vi "2D experiment mouse.vi"() -> ()   [LabVIEW 2011]
uses:
  <vilib>/Platform/TimedLoop/XDataNode/timing_clust.ctl
  <vilib>/Platform/TimedLoop/XDataNode/nitl_modes.ctl
  <vilib>/Platform/TimedLoop/XDataNode/wakeup.ctl
  <vilib>/Utility/cursorutil.llb/Set Cursor (Cursor ID).vi
  <vilib>/Utility/inputDevices.llb/closeMouse.vi
  <vilib>/Utility/inputDevices.llb/mouseAcquire.vi
  <vilib>/Utility/file.llb/Write To Spreadsheet File (DBL).vi
  <vilib>/Utility/file.llb/Write To Spreadsheet File (I64).vi
  <vilib>/Platform/TimedLoop/XDataNode/XDataNode.xnode
  User32.dll
  <vilib>/Platform/TimedLoop/XDataNode/XDNodeRunTimeDep.lvlib
panel:
  out "initial time":u32
  out "XY Graph":cluster{"Y":dbl[], "Y":dbl[]}[](graph)
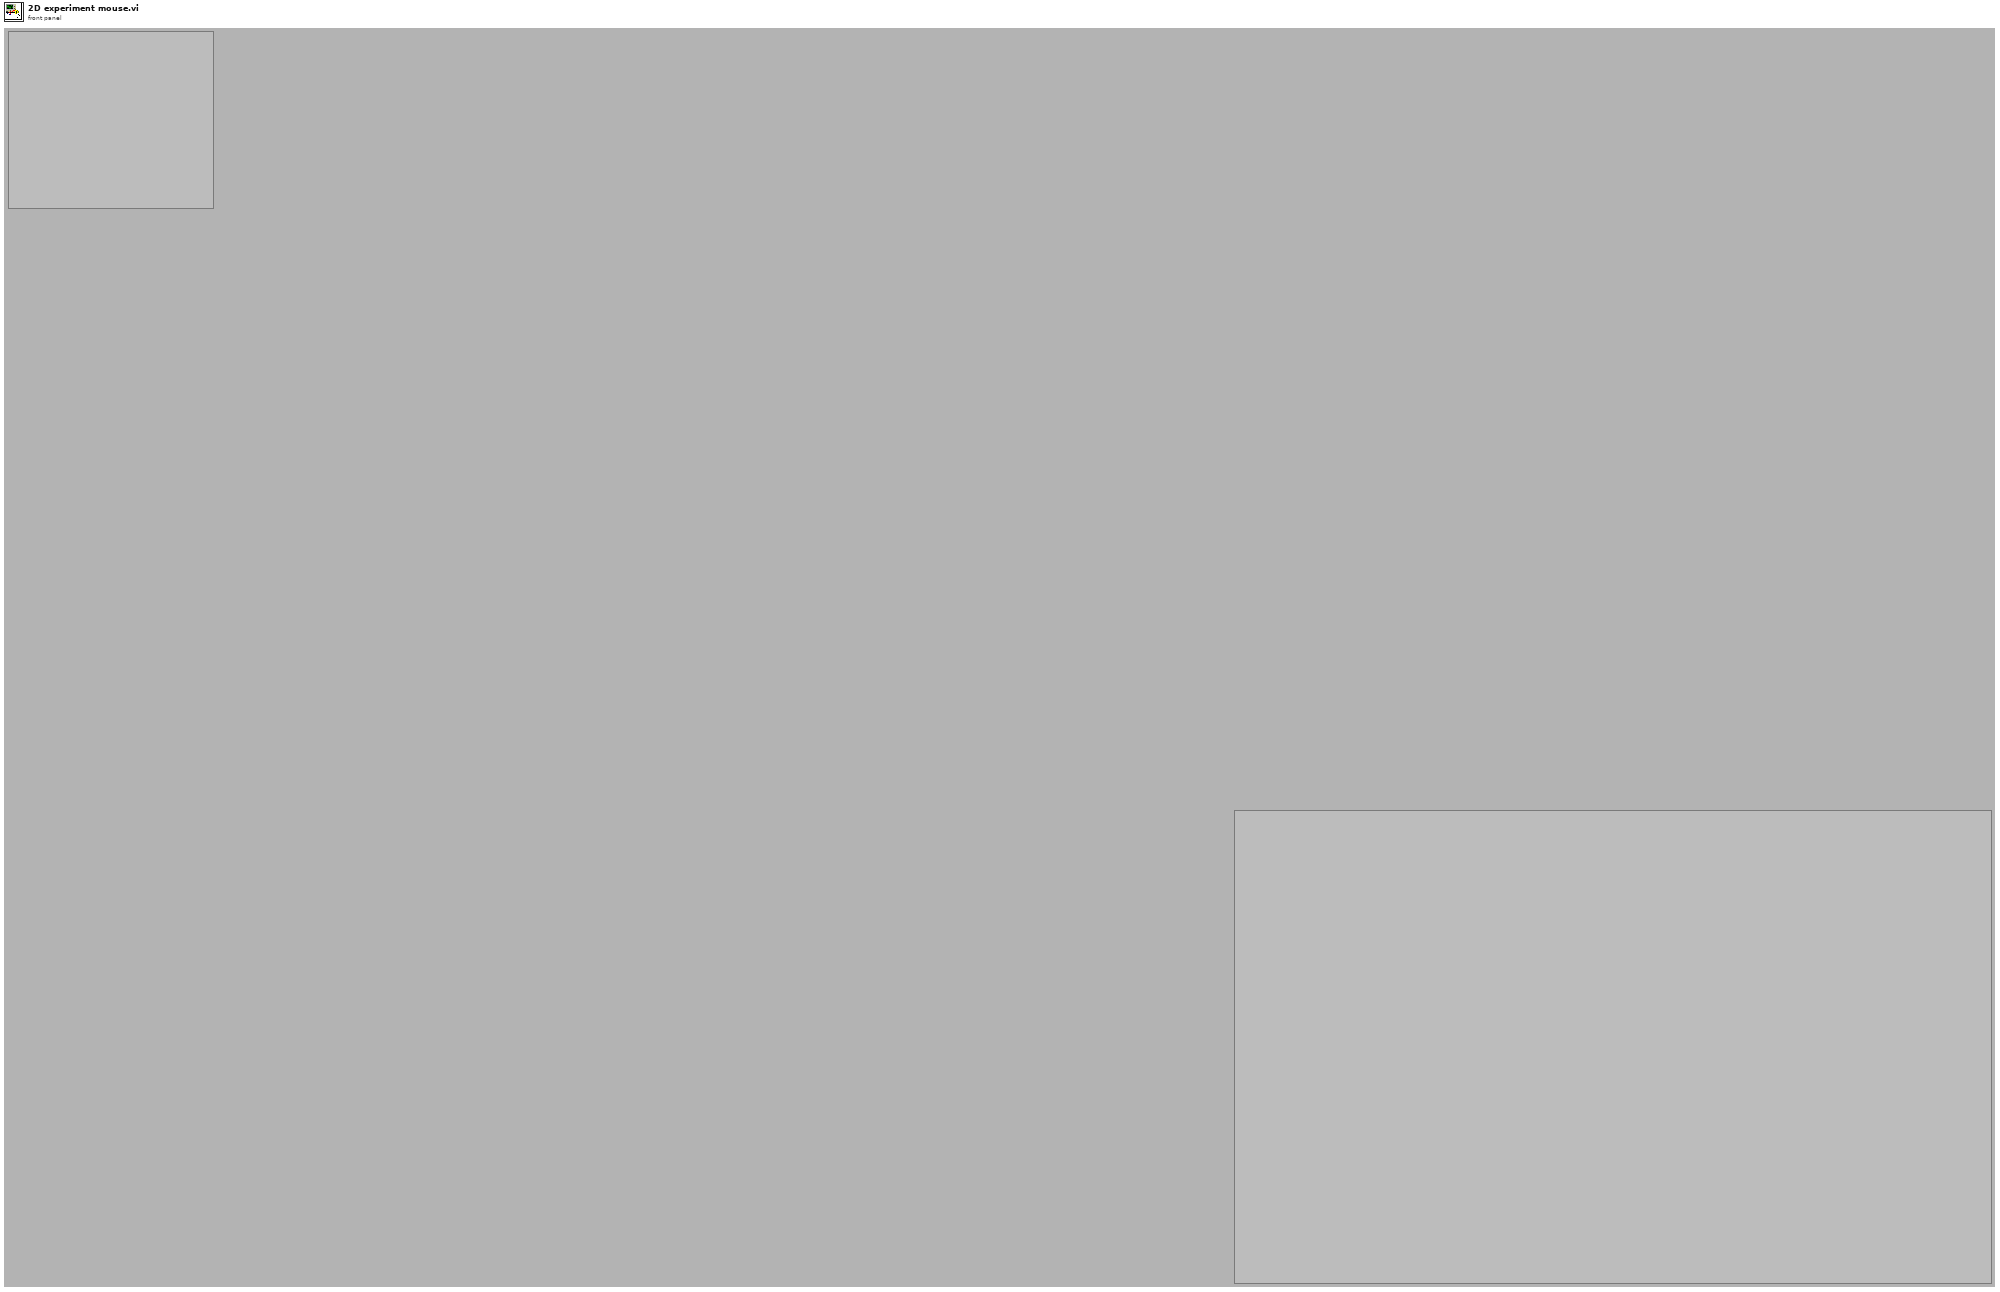
[diagram p1: front panel]
types:
  T1 = enum16{"open", "replace", "create", "open or create", "replace or create", "replace or create with confirmation"}
  T2 = typedef "XDNodeRunTimeDep.lvlib/timing_clust.ctl" = cluster{"Expected End [f-1]":u64, "Actual End [f-1]":u64, "Finished Late? [f-1]":bool, "Expected End [i-1]":u64, "Actual End [i-1]":u64, "Finished Late? [i-1]":bool, "Expected Start [i]":u64, "Actual Start [i]":u64, "Expected Start [f]":u64, "Actual Start [f]":u64, "Source Name":string, "Structure Name":string, "Period":i64, "Deadline":i64, "Offset":i64, "Start":i64, "Priority":i32, "Timeout":i32, "Mode":T3, "Wakeup Reason":T4, "Error":errorcluster, "Source Type":string, "Secondary Source Type":string, "Global End Time":u64, "Global Start Time":u64, "Frame Duration":u64, "Iteration Duration":u64, "Assigned CPU":i32, "I/O Scan Engine Mode":u32}
  T3 = typedef "XDNodeRunTimeDep.lvlib/nitl_modes.ctl" = enum32{"No Change", "Process missed periods, maintain original phase", "Discard missed periods, maintain original phase", "Process missed periods, ignore original phase", "Discard missed periods, ignore original phase"}
  T4 = typedef "XDNodeRunTimeDep.lvlib/wakeup.ctl" = enum32{"Normal", "Aborted", "Asynchronous wakeup", "Timing source error", "Timed loop error", "Timeout"}
  T5 = typedef "LVAllMonitorsDisplayTypeDef.ctl" = cluster{"Bounds":cluster{"Left":i16, "Top":i16, "Right":i16, "Bottom":i16}, "Depth":i16}[]
  T6 = cluster{"Bounds":cluster{"Left":i16, "Top":i16, "Right":i16, "Bottom":i16}, "Depth":i16}
  T7 = cluster{"Left":i16, "Top":i16, "Right":i16, "Bottom":i16}
  T8 = cluster{"Horizontal":i32, "Vertical":i32, "Scrolling":i32}
  T9 = cluster{"button 1":bool, "button 2":bool, "button 3":bool, "button 4":bool}
  T10 = cluster{"Radius":dbl, "x0":dbl, "y0":dbl, "D":dbl, bool}
  T11 = typedef "LVPoint32TypeDef.ctl" = cluster{"Horizontal":i32, "Vertical":i32}
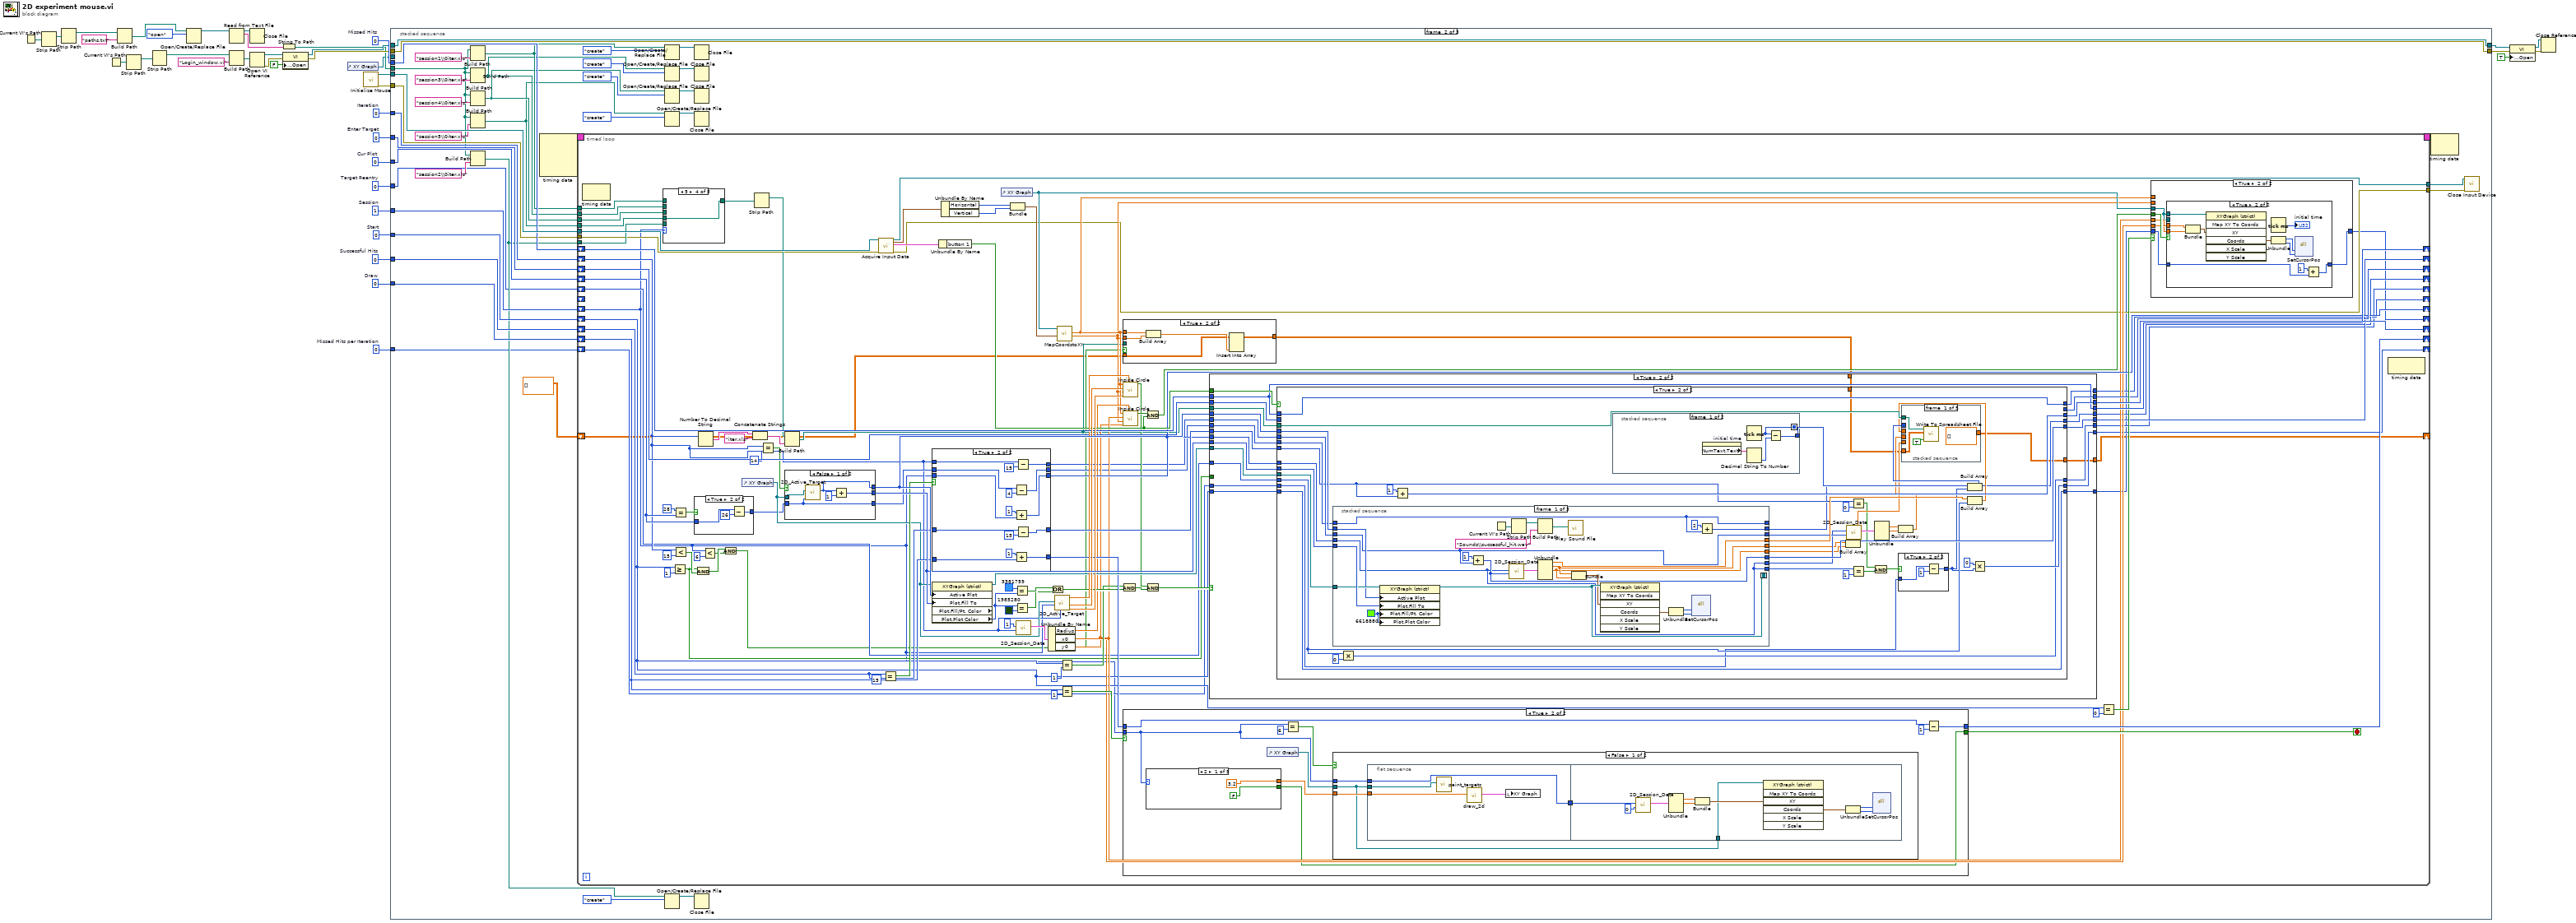
[diagram p0: block diagram]
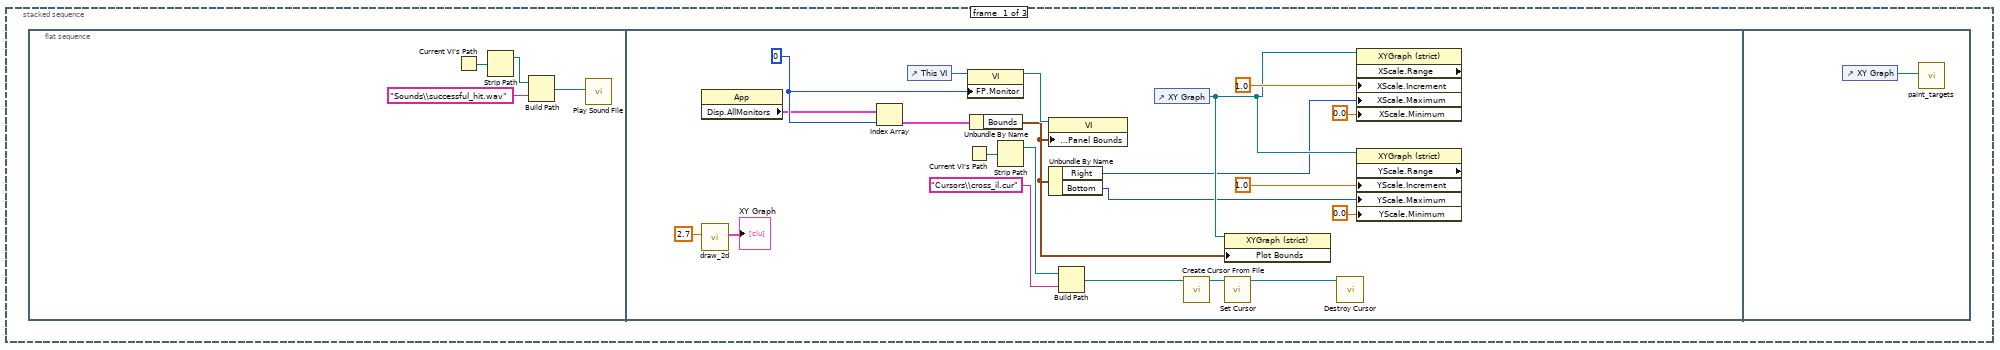
[diagram p2: hidden frame]
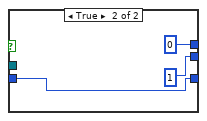
[diagram p8: hidden frame]
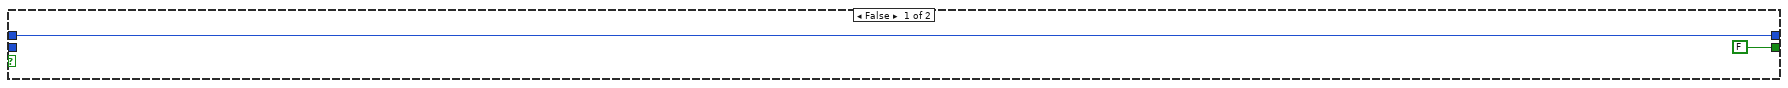
[diagram p10: hidden frame]
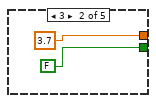
[diagram p12: hidden frame]
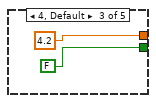
[diagram p13: hidden frame]
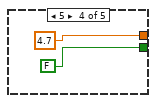
[diagram p14: hidden frame]
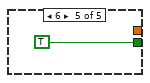
[diagram p15: hidden frame]
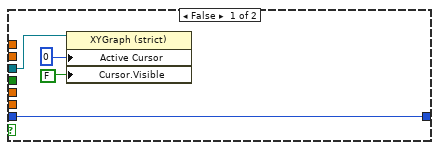
[diagram p16: hidden frame]
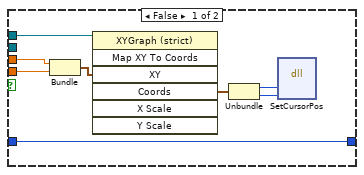
[diagram p17: hidden frame]
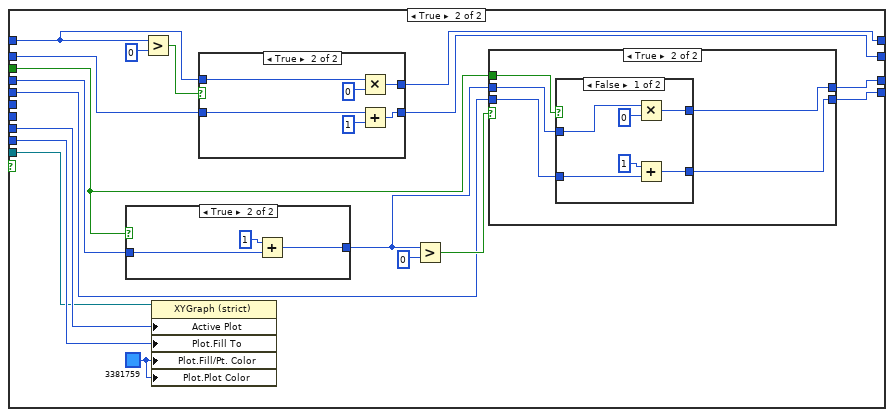
[diagram p20: hidden frame]
diagram:
  w1 = 0  # Target Reentry
  w2 = 0  # Missed Hits per Iteration
  w30 = 0  # Iteration
  w31 = 0  # Cur Plot
  w33 = 0  # Start
  w34 = 0  # Draw
  w35 = 1  # Session
  w36 = 0  # Successful Hits
  w37 = 0  # Missed Hits
  w38 = 0  # Enter Target
  n1 = Current VI's Path() -> (path=w11:path)
  n2 = Strip Path(path=w11) -> (stripped path=w6:path)  [unwired: 1 out]
  n3 = Strip Path(path=w6) -> (stripped path=w5:path)  [unwired: 1 out]
  n4 = Current VI's Path() -> (path=w26:path)
  n5 = Build Path(base path=w5, name or relative path="paths.txt") -> (appended path=w10:path)
  n6 = Strip Path(path=w26) -> (stripped path=w21:path)  [unwired: 1 out]
  n7 = Strip Path(path=w21) -> (stripped path=w20:path)  [unwired: 1 out]
  n8 = Open/Create/Replace File(file path (use dialog)=w10, operation (0:open)=T1."open") -> (refnum out=w13:refnum<file>)  [unwired: 4 in, 2 out]
  n9 = Read from Text File(file (use dialog)=w13) -> (refnum out=w14:refnum<file>, text=w12:string)  [unwired: 3 in, 2 out]
  n10 = Build Path(base path=w20, name or relative path="Login_window.vi") -> (appended path=w24:path)
  n11 = Close File(refnum=w14) -> ()  [unwired: 1 in, 2 out]
  n12 = Open VI Reference(vi path=w24) -> (vi reference=w29:refnum<vi>, error out=w28:errorcluster)  [unwired: 5 in]
  n13 = String To Path(string=w12) -> (path=w7:path)
  n14 = property class="VI"(reference=w29, error in=w28, "Front Panel Window:Open"=FALSE) -> (reference out=w23:refnum<vi>, error out=w22:errorcluster)
  n15 = control-ref of="XY Graph"() -> (w4:refnum<vi>)
  n16 = call <vilib>:"Initialize Mouse.vi"() -> ("error out"=w3:errorcluster, "device ID"=w32:refnum<k1>)  [unwired: 10 in]
  n17 = stacked-sequence {
    tunnel: w32 -> [_ w104 _]
    tunnel: w36 -> [_ w103 _]
    tunnel: w37 -> [_ w102 _]
    tunnel: w35 -> [_ w98 _]
    tunnel: w33 -> [_ w101 _]
    tunnel: w34 -> [_ w100 _]
    tunnel: w38 -> [_ w99 _]
    tunnel: w31 -> [_ w97 _]
    tunnel: w30 -> [_ w96 _]
    tunnel: w23 -> [_ w93 _]
    tunnel: w22 -> [_ w92 _]
    tunnel: [_ w93 _] -> w16
    tunnel: [_ w92 _] -> w15
    tunnel: w7 -> [_ w72 _]
    tunnel: w4 -> [_ _ w536]
    tunnel: w3 -> [_ w78 _]
    tunnel: w2 -> [_ w76 _]
    tunnel: w1 -> [_ w75 _]
    frame #0 {
      n18 = flat-sequence {
        frame #0 {
          n19 = Current VI's Path() -> (path=w40:path)
          n20 = Strip Path(path=w40) -> (stripped path=w41:path)  [unwired: 1 out]
          n21 = Build Path(base path=w41, name or relative path="Sounds\\successful_hit.wav") -> (appended path=w39:path)
          n22 = call <vilib>:"Play Sound File.vi"("path"=w39) -> ()  [unwired: 9 in, 2 out]
        }
        frame #1 {
          w59 = u16 0 ("Front Panel Window:Monitor")
          n23 = property class="App"() -> ("Disp.AllMonitors"=w58:T5)  [unwired: 2 in, 2 out]
          n24 = call "draw_2d.vi"("ID"=2.7) -> ("appended array"=→"XY Graph":cluster{dbl[], dbl[]}[])  [unwired: 10 in]
          n25 = Index Array(array=w58, index=w59) -> (element=w60:T6)
          n26 = control-ref of="This VI"() -> (w61:refnum<vi>)
          n27 = Current VI's Path() -> (path=w50:path)
          n28 = property class="VI"(reference=w61, "FP.Monitor"=w59) -> (reference out=w57:refnum<vi>)  [unwired: 1 in, 1 out]
          n29 = Unbundle By Name(w60) -> ("Bounds"=w56:T7)
          n30 = Strip Path(path=w50) -> (stripped path=w49:path)  [unwired: 1 out]
          n31 = property class="VI"(reference=w57, "Front Panel Window:Panel Bounds"=w56) -> ()  [unwired: 1 in, 2 out]
          n32 = Unbundle By Name(w56) -> ("Right"=w44:i16, "Bottom"=w43:i16)
          n33 = Build Path(base path=w49, name or relative path="Cursors\\cross_il.cur") -> (appended path=w47:path)
          n34 = control-ref of="XY Graph"() -> (w51:refnum<vi>)
          n35 = call <vilib>:"Create Cursor From File.vi"("cursor file"=w47) -> ("cursor ID"=w46:refnum<k1>)  [unwired: 9 in, 1 out]
          n36 = property on="Property Node" class="XYGraph (strict)"(reference=w51, "Plot Bounds"=w56) -> ()  [unwired: 1 in, 2 out]
          n37 = call-poly <vilib>:"Set Cursor.vi"("cursor ID"=w46) -> ("previous cursor ID"=w45:refnum<k1>)  [unwired: 9 in, 1 out]
          n38 = call <vilib>:"Destroy Cursor.vi"("cursor ID"=w45) -> ()  [unwired: 9 in, 1 out]
          n39 = property on="Property Node" class="XYGraph (strict)" props=["XScale", "Range", "XScale", "Increment", "XScale", "Maximum", "XScale", "Minimum"](reference=w51, "XScale.Increment"=1.0 ("X Scale.Range:Increment"), "XScale.Maximum"=w44, "XScale.Minimum"=0.0 ("X Scale.Range:Minimum")) -> ()  [unwired: 1 in, 3 out]
          n40 = property on="Property Node" class="XYGraph (strict)" props=["YScale", "Range", "YScale", "Increment", "YScale", "Maximum", "YScale", "Minimum"](reference=w51, "YScale.Increment"=1.0 ("Y Scale.Range:Increment"), "YScale.Maximum"=w43, "YScale.Minimum"=0.0 ("Y Scale.Range:Minimum")) -> ()  [unwired: 1 in, 3 out]
        }
        frame #2 {
          n41 = control-ref of="XY Graph"() -> (w64:refnum<vi>)
          n42 = call "paint_targets.vi"("XYGraph Refnum"=w64) -> ()  [unwired: 11 in]
        }
      }
    }
    frame #1 {
      n43 = Build Path(base path=w72, name or relative path="session1\\0iter.xls") -> (appended path=w86:path)
      n44 = Build Path(base path=w72, name or relative path="session3\\0iter.xls") -> (appended path=w80:path)
      n45 = Build Path(base path=w72, name or relative path="session4\\0iter.xls") -> (appended path=w69:path)
      n46 = Build Path(base path=w72, name or relative path="session5\\0iter.xls") -> (appended path=w66:path)
      n47 = Build Path(base path=w72, name or relative path="session2\\0iter.xls") -> (appended path=w83:path)
      n48 = node-c288() -> (w95:T2)  [unwired: 4 in]
      n49 = timed-loop {
        tunnel: w104 -> [w193]
        tunnel: [w192] -> w79
        shift-right: [w191] -> _
        shift-left: w103 -> [w176]
        shift-right: [w189] -> _
        shift-left: w102 -> [w190]
        shift-right: [w168] -> _
        shift-left: w98 -> [w113]
        shift-right: [w115] -> _
        shift-left: w101 -> [w134]
        shift-right: [w173] -> _
        shift-left: w100 -> [w174]
        shift-right: [w169] -> _
        shift-left: w99 -> [w170]
        shift-right: [w151] -> _
        shift-left: w96 -> [w125]
        shift-right: [w150] -> _
        shift-left: w97 -> [w147]
        timing: w95 -> [_]
        timing-out: [_] -> w94
        tunnel: w86 -> [w140]
        tunnel: w83 -> [w139]
        tunnel: w80 -> [w138]
        shift-right: [w127] -> _
        shift-left: _ -> [_]
        tunnel: w78 -> [w123]
        tunnel: [w122] -> w77
        shift-right: [w120] -> _
        shift-left: w76 -> [w121]
        shift-right: [w117] -> _
        shift-left: w75 -> [w119]
        tunnel: w69 -> [w109]
        tunnel: w66 -> [w108]
        shift-right: [w105] -> _
        shift-left: dbl[][] [] -> [w107]
        stop <- w162 stop-if-true
        n50 = node-c288() -> ()  [unwired: 1 in, 1 out]
        n51 = case shown="5" w113 {
          tunnel: w140 -> [_ _ _ _ w214]
          tunnel: [w210 w211 w212 w213 w214] -> w133
          tunnel: w139 -> [w210 _ _ _ _]
          tunnel: w138 -> [_ w211 _ _ _]
          tunnel: w109 -> [_ _ w212 _ _]
          tunnel: w108 -> [_ _ _ w213 _]
          frame 2 {
          }
          frame 3 {
          }
          frame 4 {
          }
          frame 5 {
          }
          frame 1, Default {
          }
        }
        n52 = Greater Or Equal?(x=w134, y=1) -> (x >= y?=w118:bool)
        n53 = Equal?(x=28, y=w147) -> (x = y?=w148:bool)
        n54 = Less?(x=w125, y=15) -> (x < y?=w124:bool)
        n55 = case shown="True" w148 {
          tunnel: w147 -> [w225 w228]
          tunnel: [w225 w226] -> w146
          frame False {
          }
          frame True {
            n56 = Subtract(x=w228, y=26) -> (x-y=w226:i32)
          }
        }
        n57 = And(x=w118, y=w124) -> (x .and. y?=w114:bool)
        n58 = Number To Decimal String(number=w125) -> (decimal integer string=w129:string)  [unwired: 1 in]
        n59 = Less?(x=w113, y=6) -> (x < y?=w111:bool)
        n60 = And(x=w114, y=w111) -> (x .and. y?=w110:bool)
        n61 = control-ref of="XY Graph"() -> (w156:refnum<vi>)
        n62 = Concatenate Strings(w129, "iter.xls" ("name or relative path")) -> (w131:string)
        n63 = Strip Path(path=w133) -> (stripped path=w130:path)  [unwired: 1 out]
        n64 = Equal?(x=w125, y=14) -> (x = y?=w144:bool)
        n65 = Build Path(base path=w130, name or relative path=w131) -> (appended path=w128:path)
        n66 = case shown="False" w144 {
          tunnel: [w220 u32 0 ("Active Plot")] -> w198
          tunnel: [w219 u32 1] -> w197
          tunnel: w156 -> [w218 _]
          tunnel: w146 -> [w217 w222]
          tunnel: [w217 w222] -> w143
          frame False {
            n67 = call "2D_Active_Target.vi"("Active Plot"=w217, "XYGraph Refnum"=w218) -> ("Active Plot"=w220:u32)  [unwired: 6 in, 3 out]
            n68 = Add(x=w220, y=u32 1) -> (x+y=w219:u32)
          }
          frame True {
          }
        }
        n69 = call-poly <vilib>:"Acquire Input Data.vi"("device ID"=w193, "error in (no error)"=w123) -> ("device ID"=w192:refnum<k1>, "axis info"=w155:T8, "button info"=w194:T9, "error out"=w122:errorcluster)  [unwired: 1 in, 13 out]
        n70 = Equal?(x=w176, y=15) -> (x = y?=w187:bool)
        n71 = case shown="True" w187 {
          tunnel: w176 -> [w300 w315]
          tunnel: [w300 w314] -> w186
          tunnel: w113 -> [w299 w313]
          tunnel: [w299 w311] -> w168
          tunnel: w174 -> [w298 w310]
          tunnel: [w298 w308] -> w172
          tunnel: w143 -> [w297 w307]
          tunnel: [w297 w305] -> w142
          tunnel: w125 -> [w296 w304]
          tunnel: [w296 w302] -> w141
          frame False {
          }
          frame True {
            n72 = Subtract(x=w307, y=4) -> (x-y=w305:i32)
            n73 = Add(x=1, y=w313) -> (x+y=w311:i32)
            n74 = Add(x=1, y=w310) -> (x+y=w308:i32)
            n75 = Subtract(x=w304, y=15) -> (x-y=w302:i32)
            n76 = Subtract(x=w315, y=15) -> (x-y=w314:i32)
          }
        }
        n77 = property on="Property Node" class="XYGraph (strict)" props=["Active Plot", "Plot", "Fill To", "Plot", "Fill/Pt. Color", "Plot", "Plot Color"](reference=w156, "Active Plot"=w198, "Plot.Fill To"=w197) -> (reference out=w177:refnum<vi>, "Plot.Plot Color"=w178:u32)  [unwired: 1 in, 2 out]
        n78 = Unbundle By Name(w194) -> ("button 1"=w181:bool)
        n79 = Unbundle By Name(w155) -> ("Horizontal"=w154:i32, "Vertical"=w153:i32)
        n80 = control-ref of="XY Graph"() -> (w152:refnum<vi>)
        n81 = Bundle("Horizontal"=w154, "Vertical"=w153) -> (w182:cluster{"Horizontal":i32, "Vertical":i32})  [unwired: 1 in]
        n82 = Equal?(x=u32 3381759, y=w178) -> (x = y?=w200:bool)
        n83 = Equal?(x=w178, y=u32 1985280) -> (x = y?=w199:bool)
        n84 = call "2D_Session_Data.vi"("Iteration"=w125, "Session"=1) -> ("output cluster"=w161:T10)  [unwired: 9 in]
        n85 = Unbundle By Name(w161) -> ("Radius"=w160:dbl, "x0"=w159:dbl, "y0"=w158:dbl)
        n86 = Or(x=w200, y=w199) -> (x .or. y?=w166:bool)
        n87 = call "2D_Active_Target.vi"("Iteration"=w125, "Session"=w113, "XYGraph Refnum"=w156) -> ("y0"=w195:dbl, "x0"=w196:dbl, "Radius"=w185:dbl)  [unwired: 5 in, 1 out]
        n88 = call "MapCoordstoXY.vi"("Coordinates"=w182, "XYGraph Refnum"=w152) -> ("Y(graph)"=w136:dbl, "X (graph)"=w137:dbl)  [unwired: 7 in]
        n89 = Equal?(x=w134, y=1) -> (x = y?=w164:bool)
        n90 = Equal?(x=w174, y=1) -> (x = y?=w171:bool)
        n91 = And(x=w164, y=w166) -> (x .and. y?=w163:bool)
        n92 = case shown="True" w110 {
          tunnel: w137 -> [_ w209]
          tunnel: w136 -> [_ w208]
          tunnel: w128 -> [_ _]
          tunnel: w107 -> [w204 w206]
          tunnel: [w204 w205] -> w106
          frame False {
          }
          frame True {
            n93 = Build Array(w209, w208) -> (w207:dbl[])
            n94 = Insert Into Array(array=w206, new element=w207) -> (w205:dbl[][])  [unwired: 2 in]
          }
        }
        n95 = call "Inside Circle.vi"("Radius"=w185, "y0"=w195, "y"=w136, "x0"=w196, "x"=w137) -> ("Inside Circle"=w165:bool)  [unwired: 6 in]
        n96 = call "Inside Circle.vi"("Radius"=w160, "y0"=w158, "y"=w136, "x0"=w159, "x"=w137) -> ("Inside Circle"=w180:bool)  [unwired: 6 in]
        n97 = case shown="True" w171 {
          tunnel: w113 -> [_ w231]
          tunnel: [w229 w238] -> w173
          tunnel: w172 -> [w229 w237]
          tunnel: [FALSE ("Valid") w235] -> w162
          frame False {
          }
          frame True {
            n98 = case shown="2" w231 {
              tunnel: [3.2 ("ID") 3.7 ("ID") 4.2 ("ID") 4.7 ("ID") _] -> w236
              tunnel: [FALSE FALSE FALSE FALSE TRUE] -> w235
              frame 2 {
              }
              frame 3 {
              }
              frame 4, Default {
              }
              frame 5 {
              }
              frame 6 {
              }
            }
            n99 = control-ref of="XY Graph"() -> (w232:refnum<vi>)
            n100 = Equal?(x=w231, y=6) -> (x = y?=w233:bool)
            n101 = case shown="False" w233 {
              tunnel: w236 -> [w243 _]
              tunnel: w232 -> [w240 _]
              tunnel: w231 -> [w241 _]
              frame False {
                n102 = flat-sequence {
                  tunnel: w243 -> [w246]
                  tunnel: w240 -> [w245]
                  tunnel: [w244] -> w242
                  tunnel: w241 -> [w244]
                  tunnel: w242 -> [w250]
                  tunnel: w240 -> [w248]
                  frame #0 {
                    n103 = call "paint_targets.vi"("XYGraph Refnum"=w245) -> ()  [unwired: 11 in]
                    n104 = call "draw_2d.vi"("ID"=w246) -> ("appended array"=w247:cluster{dbl[], dbl[]}[])  [unwired: 10 in]
                    n105 = local write "XY Graph"(w247) -> ()
                  }
                  frame #1 {
                    n106 = call "2D_Session_Data.vi"("Iteration"=0, "Session"=w250) -> ("output cluster"=w254:T10)  [unwired: 9 in]
                    n107 = Unbundle(w254) -> ("x0"=w253:dbl, "y0"=w251:dbl)  [unwired: 3 out]
                    n108 = Bundle("x0"=w253, "y0"=w251) -> (w252:cluster{"x0":dbl, "y0":dbl})  [unwired: 1 in]
                    n109 = invoke on="Invoke Node" class="XYGraph (strict)" method="Map XY To Coords"(reference=w248, "XY"=w252) -> ("Coords"=w257:T11)  [unwired: 5 in, 6 out]
                    n110 = Unbundle(w257) -> ("Horizontal"=w256:i32, "Vertical"=w255:i32)
                    n111 = dll-call lib="User32.dll" fn="SetCursorPos"(w256, w255) -> ()  [unwired: 6 in, 2 out]
                  }
                }
              }
              frame True {
              }
            }
            n112 = Subtract(x=w237, y=1) -> (x-y=w238:i32)
          }
        }
        n113 = And(x=w180, y=w181) -> (x .and. y?=w179:bool)
        n114 = And(x=w165, y=w163) -> (x .and. y?=w202:bool)
        n115 = case shown="True" w202 {
          tunnel: w181 -> [w325 w406]
          tunnel: w198 -> [w333 w403]
          tunnel: w197 -> [w332 w402]
          tunnel: w186 -> [w317 w405]
          tunnel: [w317 w404] -> w191
          tunnel: w190 -> [w327 w390]
          tunnel: [w323 w390] -> w189
          tunnel: w134 -> [w331 w401]
          tunnel: [w331 w400] -> w116
          tunnel: w177 -> [w330 w399]
          tunnel: w170 -> [w322 w398]
          tunnel: [_ w397] -> w169
          tunnel: w168 -> [w318 w396]
          tunnel: w141 -> [w329 w395]
          tunnel: [w329 w394] -> w151
          tunnel: w142 -> [w328 w393]
          tunnel: [w328 w392] -> w150
          tunnel: w128 -> [_ w391]
          tunnel: [w327 w389] -> w127
          tunnel: w121 -> [w326 w388]
          tunnel: [w324 w387] -> w120
          tunnel: w119 -> [w320 w386]
          tunnel: w118 -> [w321 _]
          tunnel: [w319 w385] -> w117
          tunnel: w106 -> [w316 w384]
          tunnel: [w316 w383] -> w105
          frame False {
            n116 = case shown="False" w321 {
              tunnel: w333 -> [_ w354]
              tunnel: w332 -> [_ w353]
              tunnel: w330 -> [_ w352]
              tunnel: w327 -> [w337 w351]
              tunnel: w326 -> [w336 w347]
              tunnel: w325 -> [_ w338]
              tunnel: [w336 w346] -> w324
              tunnel: [w337 w345] -> w323
              tunnel: w322 -> [w334 w342]
              tunnel: w320 -> [w335 w341]
              tunnel: [w335 w340] -> w319
              tunnel: [w334 w339] -> _
              tunnel: w318 -> [_ _]
              tunnel: w317 -> [_ _]
              frame False {
              }
              frame True {
                w355 = u32 3381759
                n117 = case shown="True" w338 {
                  tunnel: w351 -> [w379 w382]
                  tunnel: [w379 w380] -> w348
                  frame False {
                  }
                  frame True {
                    n118 = Add(x=1, y=w382) -> (x+y=w380:i32)
                  }
                }
                n119 = Greater?(x=w342, y=0) -> (0:w343:bool)
                n120 = property on="Property Node" class="XYGraph (strict)"(reference=w352, "Active Plot"=w354, "Plot.Fill To"=w353, "Plot.Fill/Pt. Color"=w355, "Plot.Plot Color"=w355) -> ()  [unwired: 1 in, 2 out]
                n121 = case shown="True" w343 {
                  tunnel: w342 -> [w356 w363]
                  tunnel: w341 -> [w357 w360]
                  tunnel: [w357 w359] -> w340
                  tunnel: [w356 w358] -> w339
                  frame False {
                  }
                  frame True {
                    n122 = Multiply(x=w363, y=0) -> (x*y=w358:i32)
                    n123 = Add(x=w360, y=1) -> (x+y=w359:i32)
                  }
                }
                n124 = Greater?(x=w348, y=0) -> (0:w349:bool)
                n125 = case shown="True" w349 {
                  tunnel: [w364 w370] -> w346
                  tunnel: [w365 w369] -> w345
                  tunnel: w348 -> [w365 w368]
                  tunnel: w347 -> [w364 w367]
                  tunnel: w338 -> [_ w366]
                  frame False {
                  }
                  frame True {
                    n126 = case shown="False" w366 {
                      tunnel: [w375 w377] -> w370
                      tunnel: [w373 w378] -> w369
                      tunnel: w368 -> [w372 w378]
                      tunnel: w367 -> [w371 w377]
                      frame False {
                        n127 = Multiply(x=w372, y=0) -> (x*y=w373:i32)
                        n128 = Add(x=1, y=w371) -> (x+y=w375:i32)
                      }
                      frame True {
                      }
                    }
                  }
                }
              }
            }
          }
          frame True {
            n129 = case shown="True" w406 {
              tunnel: w405 -> [w420 w433]
              tunnel: [w420 w458] -> w404
              tunnel: w403 -> [w419 w462]
              tunnel: w402 -> [w418 w461]
              tunnel: w401 -> [w417 w460]
              tunnel: [w417 w460] -> w400
              tunnel: w399 -> [w416 w459]
              tunnel: w398 -> [w415 _]
              tunnel: [w413 _] -> w397
              tunnel: w396 -> [_ w457]
              tunnel: w395 -> [w412 w456]
              tunnel: [w412 w455] -> w394
              tunnel: w393 -> [w411 w454]
              tunnel: [w411 w424] -> w392
              tunnel: w391 -> [_ w451]
              tunnel: w390 -> [w410 w450]
              tunnel: [w410 w450] -> w389
              tunnel: w388 -> [w409 w426]
              tunnel: [w409 w449] -> w387
              tunnel: w386 -> [w408 w446]
              tunnel: [w408 w444] -> w385
              tunnel: w384 -> [w407 w423]
              tunnel: [w407 w422] -> w383
              frame False {
                w421 = u32 1985280
                n130 = property on="Property Node" class="XYGraph (strict)"(reference=w416, "Active Plot"=w419, "Plot.Fill To"=w418, "Plot.Fill/Pt. Color"=w421, "Plot.Plot Color"=w421) -> ()  [unwired: 1 in, 2 out]
                n131 = Add(x=w415, y=1) -> (x+y=w413:i32)
              }
              frame True {
                n132 = stacked-sequence {
                  seq-local: [w510 _ _] -> [_ w519 w530]
                  tunnel: w462 -> [w509 w518 w532]
                  tunnel: w461 -> [w512 _ w531]
                  tunnel: w459 -> [w511 _ _]
                  tunnel: w457 -> [w490 _ _]
                  tunnel: w456 -> [w493 w517 _]
                  tunnel: [w495 _ _] -> w455
                  tunnel: [w503 _ _] -> _
                  tunnel: w454 -> [w503 _ _]
                  tunnel: [w501 _ _] -> w424
                  tunnel: [w494 _ _] -> w447
                  tunnel: [w493 _ _] -> w442
                  tunnel: [w490 _ _] -> w441
                  tunnel: [w492 _ _] -> w437
                  tunnel: [w491 _ _] -> w436
                  tunnel: [w490 _ _] -> w431
                  frame #0 {
                    w513 = u32 6618880
                    n133 = property on="Property Node" class="XYGraph (strict)"(reference=w511, "Active Plot"=w509, "Plot.Fill To"=w512, "Plot.Fill/Pt. Color"=w513, "Plot.Plot Color"=w513) -> (reference out=w510:refnum<vi>)  [unwired: 1 in, 1 out]
                    n134 = Add(x=1, y=w493) -> (x+y=w495:i32)
                    n135 = Current VI's Path() -> (path=w506:path)
                    n136 = call "2D_Session_Data.vi"("Iteration"=w495, "Session"=w490) -> ("output cluster"=w497:T10)  [unwired: 9 in]
                    n137 = Strip Path(path=w506) -> (stripped path=w505:path)  [unwired: 1 out]
                    n138 = Build Path(base path=w505, name or relative path="Sounds\\successful_hit.wav") -> (appended path=w507:path)
                    n139 = Unbundle(w497) -> ("Radius"=w494:dbl, "x0"=w492:dbl, "y0"=w491:dbl)  [unwired: 2 out]
                    n140 = call <vilib>:"Play Sound File.vi"("path"=w507) -> ()  [unwired: 9 in, 2 out]
                    n141 = Bundle("x0"=w492, "y0"=w491) -> (w496:cluster{"x0":dbl, "y0":dbl})  [unwired: 1 in]
                    n142 = invoke on="Invoke Node" class="XYGraph (strict)" method="Map XY To Coords"(reference=w510, "XY"=w496) -> ("Coords"=w500:T11)  [unwired: 5 in, 6 out]
                    n143 = Unbundle(w500) -> ("Horizontal"=w499:i32, "Vertical"=w498:i32)
                    n144 = dll-call lib="User32.dll" fn="SetCursorPos"(w499, w498) -> ()  [unwired: 6 in, 2 out]
                    n145 = Add(x=2, y=w503) -> (x+y=w501:i32)
                  }
                  frame #1 {
                    w521 = u32 3381759
                    n146 = Equal?(x=15, y=w517) -> (x = y?=w515:bool)
                    n147 = case shown="True" w515 {
                      tunnel: [w523 w527] -> w520
                      tunnel: w518 -> [w522 w529]
                      tunnel: [w522 w525] -> w514
                      frame False {
                        n148 = Add(x=w522, y=u32 1) -> (x+y=w523:u32)
                      }
                      frame True {
                        n149 = Subtract(x=w529, y=u32 2) -> (x-y=w525:u32)
                        n150 = Add(x=w525, y=1 ("x")) -> (x+y=w527:u32)
                      }
                    }
                    n151 = property on="Property Node" class="XYGraph (strict)"(reference=w519, "Active Plot"=w514, "Plot.Fill To"=w520, "Plot.Fill/Pt. Color"=w521, "Plot.Plot Color"=w521) -> ()  [unwired: 1 in, 2 out]
                  }
                  frame #2 {
                    w533 = u32 3223857
                    n152 = property on="Property Node" class="XYGraph (strict)"(reference=w530, "Active Plot"=w532, "Plot.Fill To"=w531, "Plot.Fill/Pt. Color"=w533, "Plot.Plot Color"=w533) -> ()  [unwired: 1 in, 2 out]
                  }
                }
                n153 = Multiply(x=w446, y=0) -> (x*y=w444:i32)
                n154 = Add(x=1, y=w433) -> (x+y=w458:i32)
                n155 = stacked-sequence {
                  seq-local: [w484 _] -> [_ w488]
                  tunnel: [w485 _] -> w452
                  frame #0 {
                    n156 = property on="initial time" class="DigNum (strict)"() -> ("NumText.Text"=w487:string)  [unwired: 2 in, 2 out]
                    n157 = Tick Count (ms)() -> (millisecond timer value=w484:u32)
                    n158 = Decimal String To Number(string=w487) -> (number=w486:i32)  [unwired: 2 in, 1 out]
                    n159 = Subtract(x=w484, y=w486) -> (x-y=w485:u32)
                  }
                  frame #1 {
                    n160 = Number To Decimal String(number=w488) -> (decimal integer string=w489:string)  [unwired: 1 in]
                    n161 = property on="initial time" class="DigNum (strict)"("NumText.Text"=w489) -> ()  [unwired: 2 in, 2 out]
                  }
                }
                n162 = Build Array(w437, w436) -> (w434:dbl[])
                n163 = call "2D_Session_Data.vi"("Iteration"=w442, "Session"=w441) -> ("output cluster"=w440:T10)  [unwired: 9 in]
                n164 = Equal?(x=w433, y=0) -> (x = y?=w429:bool)
                n165 = Equal?(x=w431, y=1) -> (x = y?=w428:bool)
                n166 = And(x=w429, y=w428) -> (x .and. y?=w427:bool)
                n167 = Unbundle(w440) -> ("x0"=w439:dbl, "y0"=w438:dbl)  [unwired: 3 out]
                n168 = Build Array(w439, w438) -> (w435:dbl[])
                n169 = case shown="True" w427 {
                  tunnel: w426 -> [w464 w466]
                  tunnel: [w464 w465] -> w425
                  frame False {
                  }
                  frame True {
                    n170 = Subtract(x=w466, y=1) -> (x-y=w465:i32)
                  }
                }
                n171 = Build Array(w452, w425) -> (w453:u32[])
                n172 = Build Array(w447, w446) -> (w443:dbl[])
                n173 = stacked-sequence {
                  tunnel: w453 -> [_ w474 _ _ _]
                  tunnel: w451 -> [w469 w472 w475 w480 w482]
                  tunnel: w443 -> [_ _ w477 _ _]
                  tunnel: w435 -> [_ _ _ w479 _]
                  tunnel: w434 -> [_ _ _ _ w483]
                  tunnel: w423 -> [w470 _ _ _ _]
                  tunnel: [dbl[][] [] _ _ _ _] -> w422
                  frame #0 {
                    n174 = call-poly <vilib>:"Write To Spreadsheet File.vi"("append to file? (new file:F)"=TRUE, "2D data"=w470, "file path (dialog if empty)"=w469) -> ()  [unwired: 5 in, 1 out]
                  }
                  frame #1 {
                    n175 = call-poly <vilib>:"Write To Spreadsheet File.vi"("append to file? (new file:F)"=TRUE, "1D data"=w474, "file path (dialog if empty)"=w472) -> ()  [unwired: 5 in, 1 out]
                  }
                  frame #2 {
                    n176 = call-poly <vilib>:"Write To Spreadsheet File.vi"("append to file? (new file:F)"=TRUE, "1D data"=w477, "file path (dialog if empty)"=w475) -> ()  [unwired: 5 in, 1 out]
                  }
                  frame #3 {
                    n177 = call-poly <vilib>:"Write To Spreadsheet File.vi"("append to file? (new file:F)"=TRUE, "1D data"=w479, "file path (dialog if empty)"=w480) -> ()  [unwired: 5 in, 1 out]
                  }
                  frame #4 {
                    n178 = call-poly <vilib>:"Write To Spreadsheet File.vi"("append to file? (new file:F)"=TRUE, "1D data"=w483, "file path (dialog if empty)"=w482) -> ()  [unwired: 5 in, 1 out]
                  }
                }
                n179 = Multiply(x=0, y=w425) -> (x*y=w449:i32)
              }
            }
          }
        }
        n180 = Equal?(x=w134, y=0) -> (x = y?=w183:bool)
        n181 = case shown="True" w183 {
          tunnel: w152 -> [w267 w271]
          tunnel: w137 -> [_ _]
          tunnel: w136 -> [_ _]
          tunnel: w179 -> [_ w276]
          tunnel: w116 -> [w270 w275]
          tunnel: [w270 w274] -> w115
          tunnel: w159 -> [_ w273]
          tunnel: w158 -> [_ w272]
          frame False {
            n182 = property on="Property Node" class="XYGraph (strict)"(reference=w267, "Active Cursor"=u32 0, "Cursor.Visible"=FALSE) -> ()  [unwired: 1 in, 2 out]
          }
          frame True {
            n183 = case shown="True" w276 {
              tunnel: w275 -> [w284 w291]
              tunnel: [w284 w290] -> w274
              tunnel: w273 -> [w279 w295]
              tunnel: w272 -> [w278 w294]
              tunnel: w271 -> [_ _]
              tunnel: w271 -> [w277 w293]
              frame False {
                n184 = Bundle("x0"=w279, "y0"=w278) -> (w281:cluster{"x0":dbl, "y0":dbl})  [unwired: 1 in]
                n185 = invoke on="Invoke Node" class="XYGraph (strict)" method="Map XY To Coords"(reference=w277, "XY"=w281) -> ("Coords"=w280:T11)  [unwired: 5 in, 6 out]
                n186 = Unbundle(w280) -> ("Horizontal"=w283:i32, "Vertical"=w282:i32)
                n187 = dll-call lib="User32.dll" fn="SetCursorPos"(w283, w282) -> ()  [unwired: 6 in, 2 out]
              }
              frame True {
                n188 = Bundle("x0"=w295, "y0"=w294) -> (w287:cluster{"x0":dbl, "y0":dbl})  [unwired: 1 in]
                n189 = invoke on="Invoke Node" class="XYGraph (strict)" method="Map XY To Coords"(reference=w293, "XY"=w287) -> ("Coords"=w286:T11)  [unwired: 5 in, 6 out]
                n190 = Tick Count (ms)() -> (millisecond timer value=→"initial time":u32)
                n191 = Unbundle(w286) -> ("Horizontal"=w289:i32, "Vertical"=w288:i32)
                n192 = dll-call lib="User32.dll" fn="SetCursorPos"(w289, w288) -> ()  [unwired: 6 in, 2 out]
                n193 = Add(x=1, y=w291) -> (x+y=w290:i32)
              }
            }
          }
        }
        n194 = node-c288() -> ()  [unwired: 1 in, 1 out]
      }
      n195 = Open/Create/Replace File(file path (use dialog)=w86, operation (0:open)=T1."create") -> (refnum out=w88:refnum<file>)  [unwired: 4 in, 2 out]
      n196 = Open/Create/Replace File(file path (use dialog)=w80, operation (0:open)=T1."create") -> (refnum out=w82:refnum<file>)  [unwired: 4 in, 2 out]
      n197 = Open/Create/Replace File(file path (use dialog)=w69, operation (0:open)=T1."create") -> (refnum out=w70:refnum<file>)  [unwired: 4 in, 2 out]
      n198 = Open/Create/Replace File(file path (use dialog)=w66, operation (0:open)=T1."create") -> (refnum out=w67:refnum<file>)  [unwired: 4 in, 2 out]
      n199 = Open/Create/Replace File(file path (use dialog)=w83, operation (0:open)=T1."create") -> (refnum out=w85:refnum<file>)  [unwired: 4 in, 2 out]
      n200 = Close File(refnum=w88) -> ()  [unwired: 1 in, 2 out]
      n201 = Close File(refnum=w82) -> ()  [unwired: 1 in, 2 out]
      n202 = Close File(refnum=w70) -> ()  [unwired: 1 in, 2 out]
      n203 = Close File(refnum=w67) -> ()  [unwired: 1 in, 2 out]
      n204 = Close File(refnum=w85) -> ()  [unwired: 1 in, 2 out]
      n205 = node-c288(w94) -> ()  [unwired: 1 out]
      n206 = call-poly <vilib>:"Close Input Device.vi"("error in (no error)"=w77, "device ID"=w79) -> ()  [unwired: 8 in, 1 out]
    }
    frame #2 {
      n207 = call "finish.vi"("XYGraph Refnum"=w536) -> ()  [unwired: 11 in]
      n208 = call "Time Delay3"() -> ()  [unwired: 11 in, 1 out]
    }
  }
  n209 = property class="VI"(reference=w16, error in=w15, "Front Panel Window:Open"=TRUE) -> (reference out=w19:refnum<vi>, error out=w18:errorcluster)
  n210 = Close Reference(reference=w19, error in (no error)=w18) -> ()  [unwired: 1 out]
